vi "Write DO.vi"(8 "error in (no error)":errorcluster, 9 "DO Value":bool[](array[boolean]), 11 "PXI 6515 in":refnum<class "PXI 6515.lvclass">) -> (0 "error out":errorcluster, 3 "PXI 6515 out":refnum<class "PXI 6515.lvclass">)   [LabVIEW 2021, in "DAQ IO.lvlib" / "PXI 6515.lvclass"]
uses:
  PXI 6515.lvclass
  PXI 6515.lvclass/PXI 6515.ctl
  <vilib>/DAQmx/write.llb/DAQmx Write (Digital 1D Bool NChan 1Samp 1Line).vi
  <vilib>/DAQmx/miscellaneous.llb/DAQmx Fill In Error Info.vi
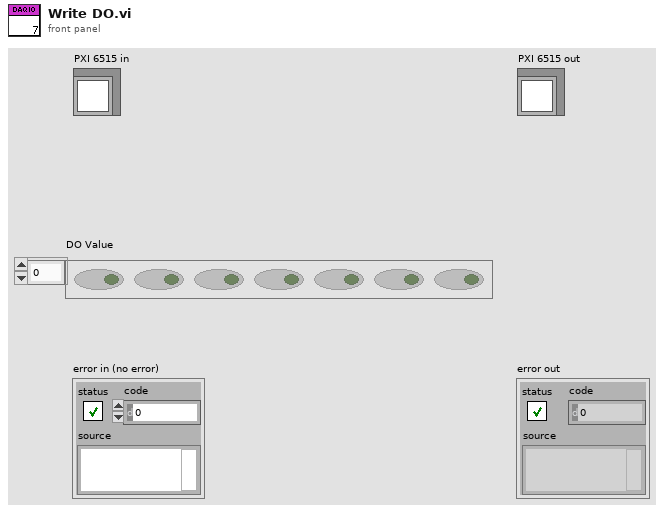
[diagram p1: front panel]
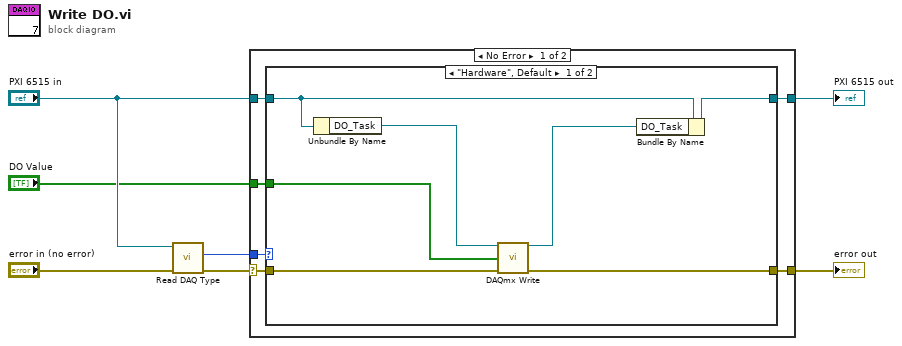
[diagram p0: block diagram]
diagram:
  n1 = call-dynamic "Read DAQ Type.vi"("error in (no error)"="error in (no error)", "PXI 6515 in"="PXI 6515 in") -> ("error out"=w6:errorcluster, "DAQ Type"=w5:enum16{"Hardware", "Simulation"})  [unwired: 7 in, 1 out]
  n2 = case shown="No Error" w6 {
    selector: w6 -> [w13 w23]
    tunnel: w5 -> [w12 _]
    tunnel: "PXI 6515 in" -> [w11 w24]
    tunnel: [w10 w24] -> w3
    tunnel: "DO Value" -> [w9 _]
    tunnel: [w8 w23] -> w1
    frame No Error {
      n3 = case shown="\"Hardware\", Default" w12 {
        tunnel: w13 -> [w20 w21]
        tunnel: w11 -> [w19 w22]
        tunnel: [w17 w22] -> w10
        tunnel: w9 -> [w18 _]
        tunnel: [w16 w21] -> w8
        frame "Hardware", Default {
          n4 = Unbundle By Name(w19) -> ("DO_Task"=w15:refnum<k21>)
          n5 = call-poly <vilib>:"DAQmx Write.vi"("task/channels in"=w15, "data"=w18, "error in"=w20) -> ("task out"=w14:refnum<k21>, "error out"=w16:errorcluster)  [unwired: 10 in, 1 out]
          n6 = Bundle By Name(cluster=w19, "DO_Task"=w14) -> (w17:refnum<class "PXI 6515.lvclass">)
        }
        frame "Simulation" {
        }
      }
    }
    frame Error {
    }
  }
  "error out" <- w1
  "PXI 6515 out" <- w3
